vi "Set Operation.vi"(7 "PW":i16=100, 8 "error in (no error)":errorcluster, 9 "BLV":dbl=2.0 format="%#_13g", 10 "WLV":dbl=3.5 format="%#_13g", 11 "instrument handle":refnum<k15>="PXI1Slot2 (16)") -> (0 "error out":errorcluster, 3 "instrument handle out":refnum<k15>="PXI1Slot2 (16)")   [LabVIEW 2018]
uses:
  <instrlib>/niDigital/niDigital.llb/niDigital Burst Pattern (Burst Only).vi
  Globals.vi
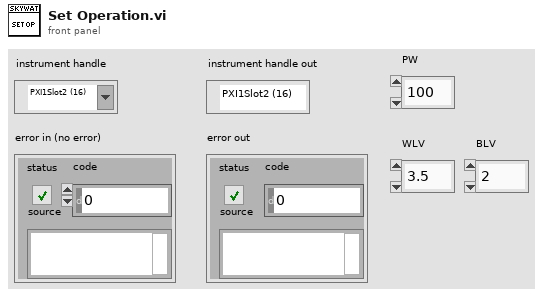
[diagram p1: front panel]
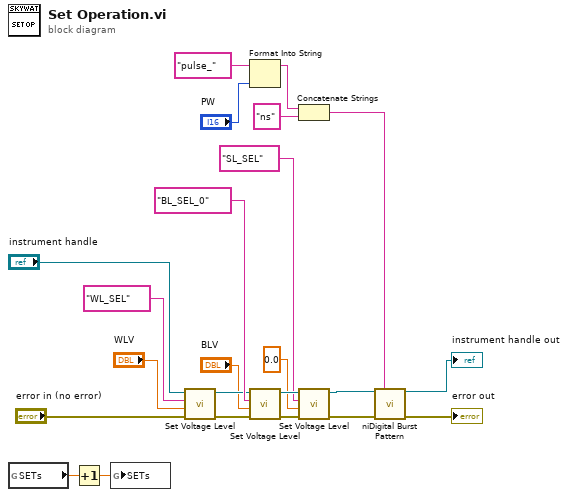
[diagram p0: block diagram]
diagram:
  n1 = global read "Globals.vi" "SETs"() -> (w4:dbl)
  n2 = Increment(x=w4) -> (x+1=w3:dbl)
  n3 = global write "Globals.vi" "SETs"(w3) -> ()
  n4 = call "Set Voltage Level.vi"("error in (no error)"="error in (no error)", "level (V)"="WLV", "channel list"="WL_SEL", "instrument handle"="instrument handle") -> ("error out"=w17:errorcluster, "instrument handle out"=w18:refnum<k15>)  [unwired: 6 in]
  n5 = Format Into String(initial string="pulse_" ("start label"), "PW") -> (resulting string=w8:string)  [unwired: 2 in, 1 out]
  n6 = call "Set Voltage Level.vi"("error in (no error)"=w17, "level (V)"="BLV", "channel list"="BL_SEL_0", "instrument handle"=w18) -> ("error out"=w16:errorcluster, "instrument handle out"=w19:refnum<k15>)  [unwired: 6 in]
  n7 = Concatenate Strings(w8, "ns" ("string")) -> (w6:string)
  n8 = call "Set Voltage Level.vi"("error in (no error)"=w16, "level (V)"=0.0, "channel list"="SL_SEL", "instrument handle"=w19) -> ("error out"=w11:errorcluster, "instrument handle out"=w13:refnum<k15>)  [unwired: 6 in]
  n9 = call-poly <instrlib>:"niDigital Burst Pattern.vi"("instrument handle"=w13, "start label"=w6, "error in"=w11) -> ("instrument handle out"=→"instrument handle out":refnum<k15>, "error out"=→"error out":errorcluster)  [unwired: 11 in]
